vi "Enable.vi"(8 "error in (no error)":errorcluster, 11 "Node Ptr":T1 format="%.0x") -> (0 "error out":errorcluster)   [LabVIEW 2026, in "Nominal Core Streaming System Explorer.lvlib"]
uses:
  Nominal Core Streaming System Explorer.lvlib
  <vilib>/NI VeriStand/Custom Device API/Custom Device Item Ref.ctl
  <vilib>/NI VeriStand/Custom Device API/Custom Device API.lvlib
panel:
  in  "initial state":bool
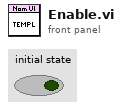
[diagram p1: front panel]
types:
  T1 = typedef "Custom Device API.lvlib/Custom Device Item Ref.ctl" = u64
  T2 = typedef "Custom Device API.lvlib/Custom Device Channel.ctl" = cluster{"Type":T3, "Units":string, "Default Value":dbl, "Faultable":bool, "Scalable":bool}
  T3 = typedef "Custom Device API.lvlib/Custom Device Channel Type.ctl" = enum16{"Input", "Output"}
  T4 = typedef "Custom Device API.lvlib/Custom Device Commands.ctl" = enum16{"Default", "Item renamed", "Shutdown", "Dynamic button pressed"}
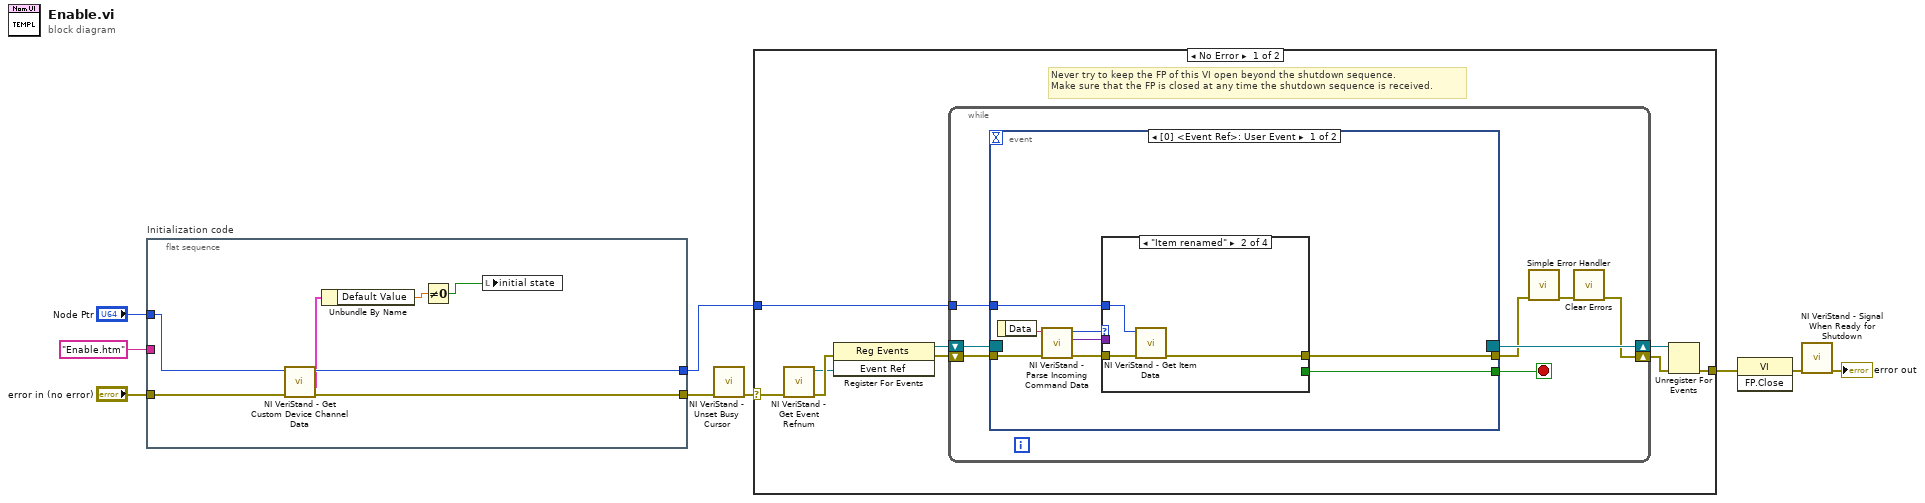
[diagram p0: block diagram]
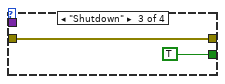
[diagram p3: hidden frame]
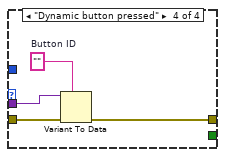
[diagram p4: hidden frame]
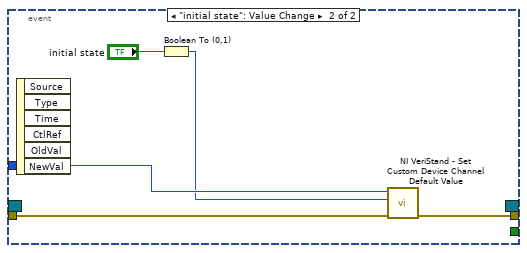
[diagram p5: hidden frame]
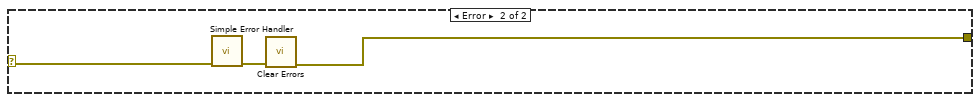
[diagram p6: hidden frame]
diagram:
  n1 = flat-sequence "Initialization code" {
    tunnel: "error in (no error)" -> [w16]
    tunnel: "Node Ptr" -> [w14]
    tunnel: [w15] -> w5
    tunnel: [w13] -> w2
    tunnel: "Enable.htm" ("CD_CHM_Section") -> [_]
    frame #0 {
      n2 = call <vilib>:"NI VeriStand - Get Custom Device Channel Data.vi"("error in (no error)"=w16, "Channel Ref in"=w14) -> ("error out"=w15:errorcluster, "Channel"=w12:T2, "Channel Ref out"=w13:T1)  [unwired: 4 in, 3 out]
      n3 = Unbundle By Name(w12) -> ("Default Value"=w11:dbl)
      n4 = Not Equal To 0?(x=w11) -> (x != 0?=w10:bool)
      n5 = local write "initial state"(w10) -> ()
    }
  }
  n6 = call <vilib>:"NI VeriStand - Unset Busy Cursor.vi"("error in (no error)"=w5) -> ("error out"=w4:errorcluster)  [unwired: 10 out]
  n7 = case shown="No Error" w4 {
    selector: w4 -> [w17 w59]
    tunnel: [w22 w57] -> w9
    tunnel: w2 -> [w18 _]
    frame No Error {
      # "Never try to keep the FP of this VI open beyond the shutdown sequence.\nMake sure that the FP is closed at any time the shutdown sequence is received."
      n8 = call <vilib>:"NI VeriStand - Get Event Refnum.vi"("error in (no error)"=w17) -> ("error out"=w25:errorcluster, "Event Ref"=w21:refnum<user-event>)  [unwired: 9 out]
      n9 = register-events(error in=w25, w21) -> (reference out=w19:refnum<event-registration>, error out=w20:errorcluster)  [unwired: 1 in]
      n10 = while {
        tunnel: w18 -> [w29]
        shift-right: [w26] -> w23
        shift-left: w20 -> [w32]
        shift-right: [w33] -> w24
        shift-left: w19 -> [w31]
        stop <- w30 stop-if-true
        n11 = event shown="[0] <Event Ref>: User Event" {
          selector: w31 -> [_ _]
          dyn-events: [_ _] -> w33
          timeout: _ -> [_ _]
          tunnel: w32 -> [w41 w55]
          tunnel: [w37 _] -> w30
          tunnel: [w36 w54] -> w28
          tunnel: w29 -> [w35 w56]
          event User Event {
            n12 = event-data() -> ("Data"=w40:string)  [unwired: 1 out]
            n13 = call <vilib>:"NI VeriStand - Parse Incoming Command Data.vi"("error in (no error)"=w41, "Incoming data"=w40) -> ("error out"=w39:errorcluster, "Outgoing data"=w34:variant, "Action"=w38:T4)  [unwired: 7 out]
            n14 = case shown="\"Item renamed\"" w38 {
              tunnel: w39 -> [w42 w45 w46 w51]
              tunnel: [_ _ TRUE _] -> w37
              tunnel: [w42 w43 w46 w48] -> w36
              tunnel: w35 -> [_ w44 _ _]
              tunnel: w34 -> [_ _ _ w50]
              frame "Default", Default {
              }
              frame "Item renamed" {
                n15 = call <vilib>:"NI VeriStand - Get Item Data.vi"("error in (no error)"=w45, "Item Ref in"=w44) -> ("error out"=w43:errorcluster)  [unwired: 9 out]
              }
              frame "Shutdown" {
              }
              frame "Dynamic button pressed" {
                w49 = ""  # Button ID
                n16 = Variant To Data(error in=w51, type=w49, Variant=w50) -> (error out=w48:errorcluster)  [unwired: 1 out]
              }
            }
          }
          event "initial state": Value Change {
            n17 = event-data() -> ()  [unwired: 7 out]
            n18 = Boolean To (0,1)(Boolean="initial state") -> (0, 1=w52:i16)
            n19 = call <vilib>:"NI VeriStand - Set Custom Device Channel Default Value.vi"("error in (no error)"=w55, "Default Value"=w52, "Channel Ref in"=w56) -> ("error out"=w54:errorcluster)  [unwired: 7 in, 1 out]
          }
        }
        n20 = call <vilib>:"Simple Error Handler.vi"("error in (no error)"=w28) -> ("error out"=w27:errorcluster)  [unwired: 1 in, 7 out]
        n21 = call <vilib>:"Clear Errors.vi"("error in (no error)"=w27) -> ("error out"=w26:errorcluster)  [unwired: 1 in, 5 out]
      }
      n22 = Unregister For Events(event registration refnum=w24, error in=w23) -> (error out=w22:errorcluster)
    }
    frame Error {
      n23 = call <vilib>:"Simple Error Handler.vi"("error in (no error)"=w59) -> ("error out"=w58:errorcluster)  [unwired: 1 in, 7 out]
      n24 = call <vilib>:"Clear Errors.vi"("error in (no error)"=w58) -> ("error out"=w57:errorcluster)  [unwired: 1 in, 5 out]
    }
  }
  n25 = invoke class="VI" method="FP.Close"(error in=w9) -> (error out=w8:errorcluster)  [unwired: 2 in, 2 out]
  n26 = call <vilib>:"NI VeriStand - Signal When Ready for Shutdown.vi"("error in (no error)"=w8) -> ("error out"=→"error out":errorcluster)  [unwired: 10 out]
